vi "Find By String.vi"(8 "error in (no error)":errorcluster, 9 "ID String Type":T1, 10 "Identification String":string, 11 "Instrument Detection in":refnum<class "Instrument Detection.lvclass">) -> (0 "error out":errorcluster, 1 "Uniquely Identified?":bool, 2 "Possible Instruments":T2[](array[typedef]), 3 "Instrument Detection out":refnum<class "Instrument Detection.lvclass">)   [LabVIEW 2020, in "Instrument Detection.lvlib" / "Instrument Detection.lvclass"]
doc: "Identify instrument by an Identification String of String Type. All found Possible Instruments are returned."
uses:
  Instrument Detection.lvclass
  Controls/Ctl_InstrumentID.ctl
  Controls/Ctl_IDStringType.ctl
  Instrument Detection.lvlib
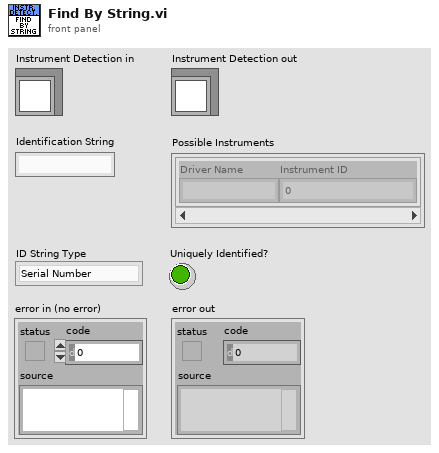
[diagram p1: front panel]
types:
  T1 = typedef "Instrument Detection.lvlib/Ctl_IDStringType.ctl" = enum16{"Serial Number", "Product Name", "Vendor Name", "Description"}
  T2 = typedef "Instrument Detection.lvlib/Ctl_InstrumentID.ctl" = cluster{"Driver Name":string, "Instrument ID":u32}
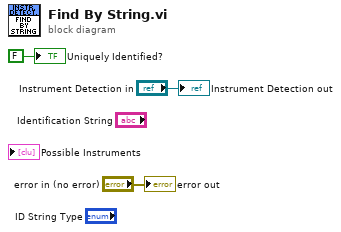
[diagram p0: block diagram]
diagram:
  "error out" <- "error in (no error)"
  "Instrument Detection out" <- "Instrument Detection in"
  "Uniquely Identified?" <- FALSE ("Found?")
